vi "2.vi"(4 "Z":bool, 5 "Y":bool, 6 "X":bool, 7 "W":bool) -> (0 "D":bool, 1 "C":bool, 2 "B":bool, 3 "A":bool)   [LabVIEW 2016]
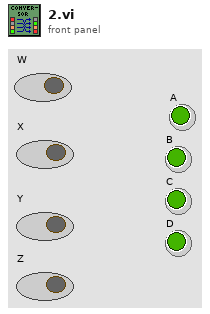
[diagram p1: front panel]
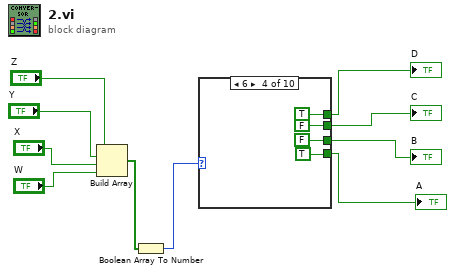
[diagram p0: block diagram]
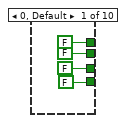
[diagram p2: hidden frame]
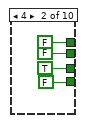
[diagram p3: hidden frame]
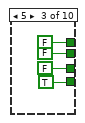
[diagram p4: hidden frame]
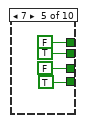
[diagram p5: hidden frame]
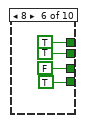
[diagram p6: hidden frame]
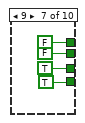
[diagram p7: hidden frame]
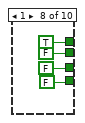
[diagram p8: hidden frame]
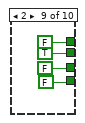
[diagram p9: hidden frame]
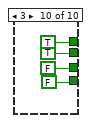
[diagram p10: hidden frame]
diagram:
  n1 = Build Array("Z", "Y", "X", "W") -> (w5:bool[])
  n2 = Boolean Array To Number(Boolean array=w5) -> (number=w10:u32)
  n3 = case shown="6" w10 {
    tunnel: [FALSE FALSE FALSE TRUE FALSE TRUE FALSE TRUE FALSE TRUE] -> w9
    tunnel: [FALSE FALSE FALSE FALSE TRUE TRUE FALSE FALSE TRUE TRUE] -> w8
    tunnel: [FALSE TRUE FALSE FALSE FALSE FALSE TRUE FALSE FALSE FALSE] -> w6
    tunnel: [FALSE FALSE TRUE TRUE TRUE TRUE TRUE FALSE FALSE FALSE] -> w7
    frame 0, Default {
    }
    frame 4 {
    }
    frame 5 {
    }
    frame 6 {
    }
    frame 7 {
    }
    frame 8 {
    }
    frame 9 {
    }
    frame 1 {
    }
    frame 2 {
    }
    frame 3 {
    }
  }
  "A" <- w7
  "B" <- w6
  "C" <- w8
  "D" <- w9
